vi "Compressor Rig PC Main.vi"() -> ()   [LabVIEW 2018]
uses:
  type defs/rigStatusCluster.ctl
  type defs/UI loop data.ctl
  type defs/event data.ctl
  supporting VIs/polymorphic VIs/enqueue for message handler.vi
  supporting VIs/polymorphic VIs/enqueue for comms.vi
  supporting VIs/polymorphic VIs/enqueue for file IO.vi
  supporting VIs/polymorphic VIs/de-queue for user interface.vi
  supporting VIs/polymorphic VIs/release user interface queue.vi
  RT/Message Handler loop/FPGA commands/RT - FPGA commands.lvlib
panel:
  in  "startPulsator":bool
  out "pulsatorHome":bool caption="Home"
  out "pulsatorSpeed":i32 caption="Actual:" min=0 max=65
  in  "pulsatorSetpoint":i32 caption="Target:" min=0 max=5000
  out "Interlocks":T1
  in  "openValves":bool
  in  "ballDemand":dbl caption="Ball Valve (%)" min=0.0 max=100.0 format="%_3g"
  in  "butterflyDemand":dbl=100.0 caption="Butterfly Valve (%)" min=0.0 max=100.0 format="%_3g"
  out "actualBall":dbl caption="Ball position" format="%_3f"
  out "actualButterfly":dbl caption="Butterfly position" format="%_3f"
  out "PR":dbl caption="Pressure Ratio" format="%_4f"
  out "massFlow":dbl caption="Mass Flow (kg/s)" format="%_4f"
  in  "logLimitEnabled":bool caption="limit logging"
  in  "pointLimit":u32 caption="datapoints"
  in  "timeLimit":dbl caption="log time (s)"
  in  "logData":bool
  out "speedGauge":dbl(knob) scale=0.0..75.0
  in  "targetSpeed":dbl caption="Target Speed (kRPM):" min=0.0 max=80.0 step=0.1 format="%_4g"
  in  "motorStart":bool
  out "statusCluster":T2 {"outletTemp" scale=0.0..100.0; "bearingTemp" scale=0.0..100.0; "gearboxTemp" scale=0.0..100.0}
  out "connected":bool caption="Compressor Rig Connected"
  in  "QUIT":bool
  # "Pulsator"
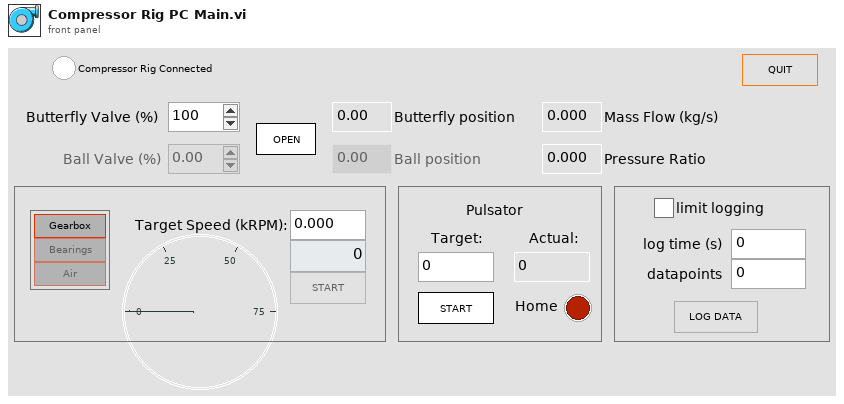
[diagram p1: front panel]
types:
  T1 = cluster{"gearboxOil":bool, "bearingOil":bool, "gearboxAir":bool}
  T2 = typedef "rigStatusCluster.ctl" = cluster{"water":bool, "airPressure":bool, "motorEnabled":bool, "oilPressure":bool, "outletTemp":dbl, "bearingTemp":dbl, "gearboxTemp":dbl}
  T3 = typedef "event data.ctl" = cluster{"menuRef":refnum<k9>, "channelConfigPath":path, "tempOffsets":dbl[]}
  T4 = typedef "UI loop data.ctl" = cluster{"params":cluster{"channelConfigPath":path, "version":string}, "vars":cluster{"tempOffsets":dbl[], "encoderFallingEdge":bool, "controlRefs":cluster{"mainVI":refnum<vi>, "menu":refnum<k9>, "motorStart":refnum<vi>, "butterfly":refnum<vi>, "ball":refnum<vi>, "speed":refnum<vi>, "logLimit":refnum<vi>, "pointLimit":refnum<vi>, "logData":refnum<vi>}}}
  T5 = typedef "message handler data.ctl" = cluster{"params":cluster{"configFileID":u32, "configFilePath":path, "channelConfigFilePath":path, "incidentLogfile":path, "controlChannels":cluster{"ballControl":u16, "butterflyControl":u16, "speedControl":u16}, "pulsatorVIPath":path, "customVIPath":path, "HowdenAir":cluster{"vent Howden":bool, "Howden%":dbl}}, "vars":cluster{"commsStatus":bool[], "controlIndex":cluster{"ballControl":u16, "butterflyControl":u16, "speedControl":u16}, "customVIRef":refnum<vi>, "Interlocks":cluster{"gearboxOil":bool, "bearingOil":bool, "gearboxAir":bool}, "motorRunning":bool, "liveDataQ":refnum<queue>[]}}
  T6 = typedef "comms loop data.ctl" = cluster{"params":cluster{"commandStream":cluster{"reader name":string, "writer name":string, "stream buffer size":i32}, "errorStream":cluster{"reader name":string, "writer name":string, "stream buffer size":i32}, "RT IP address":string, "pulserControllerIP":string}, "vars":cluster{"commandStream":refnum<k21>, "Incident logger":refnum<class "Incident logger.lvclass">, "check error scheduled message":u32, "errorStream":refnum<k21>, "watchdogScheduleID":u32, "pulsator":cluster{"pulser connection":refnum<class "Modbus Master.lvclass">, "pulserConnected":bool, "pulsatorScheduleID":u32, "pulserRunning":bool}}}
  T7 = typedef "data stream data.ctl" = cluster{"params":cluster{"Stream":cluster{"reader name":string, "RT IP address":string, "writer name":string, "stream buffer size":i32}}, "vars":cluster{"data stream":refnum<k21>}}
  T8 = typedef "data processor data.ctl" = cluster{"params":cluster{"controlFeedback":cluster{"butterflyValue":u16, "ballValue":u16, "massflow":u16, "pressureRatio":u16, "compSpeed":u16}, "DAQrate":enum16{"50 kHz", "25 kHz", "16.6 kHz", "12.5 kHz", "10 kHz", "8.33 kHz", "7.14 kHz", "6.25 kHz", "5.55 kHz", "5 kHz"}, "safetyChannels":cluster{"oilP":u16, "airP":u16, "water":u16, "channelLimit":T9[]}, "channelConfigPath":path}, "vars":cluster{"controlFeedback":cluster{"butterflyValue":u16, "ballValue":u16, "massflow":u16, "pressureRatio":u16, "compSpeed":u16}, "activeChannelNames":string[], "activeChannelUnits":string[], "offset trigger":bool, "offsets":dbl[], "activeChannelLimitIndex":u16[], "liveData":bool}}
  T9 = typedef "channelLimitControl.ctl" = cluster{"channelID":u16, "Enabled":bool, "warnValue":dbl, "limitValue":dbl, "Invert":bool, "limitAction":T10}
  T10 = typedef "limitActions.ctl" = enum16{"stop", "shutdown", "ignore"}
  T11 = typedef "file IO data.ctl" = cluster{"params":cluster{"startFolder":path, "channelConfigPath":path}, "vars":cluster{"channelConfig ":T12[], "writing":cluster{"streaming":bool, "fixedLength":bool, "pointCount":u32, "timeZero":dbl, "pointsWritten":u32, "dataRate":u16}, "channelCount":u16, "fileTarget":cluster{"Save folder":path, "Target filename":string, "file ref":refnum<file>, "pulsatorSpeed":string, "motorSpeed":string, "valvePosition":string, "torqueFilter":bool, "pulsatorRunning":bool, "motorRunning":bool}, "channels":refnum<class "Data Channel.lvclass">[]}}
  T12 = typedef "channelControl.ctl" = cluster{"index":u16, "active":bool, "channelType":T13, "module":u16, "terminal":u16, "channelName":string, "scalingMethod":T14, "scalingParameters":dbl[], "scaledUnits":string, "tempOffset":dbl}
  T13 = typedef "channelScalingTypes.ctl" = enum16{"calculation", "measurement", "scanivalve", "output", "digital"}
  T14 = typedef "scalingMethods.ctl" = enum16{"none", "linear", "thermocouple", "polynomial", "encoder", "RTD"}
  T15 = typedef "error messages data.ctl" = cluster{"params":cluster{"eg":bool}, "vars":cluster{"eg":bool}}
  T16 = cluster{"messageHandler":T5, "comms":T6, "dataStream":T7, "dataProcessor":T8, "fileIO":T11, "userInterface":T4, "errors":T15}
  T17 = typedef "Queues.ctl" = cluster{"messageHandler":refnum<queue>, "comms":refnum<queue>, "dataStream":refnum<queue>, "dataProcessor":refnum<queue>, "fileIO":refnum<queue>, "userInterface":refnum<queue>, "errors":refnum<queue>, "customCompressor":refnum<queue>}
  T18 = enum8{"Enabled", "Disabled", "Disabled and Grayed Out"}
  T19 = cluster{"actualSpeed":dbl, "butterfly":dbl, "ball":dbl, "massflow":dbl, "PR":dbl}
  T20 = typedef "eventvkey.ctl" = enum16{"ASCII", "Enter", "Return", "Shift", "Ctrl", "Alt", "Cmd", "Opt", "Caps", "NumLock", "Clear", "Break", "Up", "Down", "Left", "Right", "Insert", "Delete", "Home", "End", "PageUp", "PageDown", "Escape", "Help", "Pause", "ScrollLock", "F1", "F2", "F3", "F4", "F5", "F6", "F7", "F8", "F9", "F10", "F11", "F12", "F13", "F14", "F15", "F16", "F17", "F18", "F19", "F20", "F21", "F22", "F23", "F24", "Play", "VolumeUp", "VolumeDown", "Mute", "Two Byte Char"}
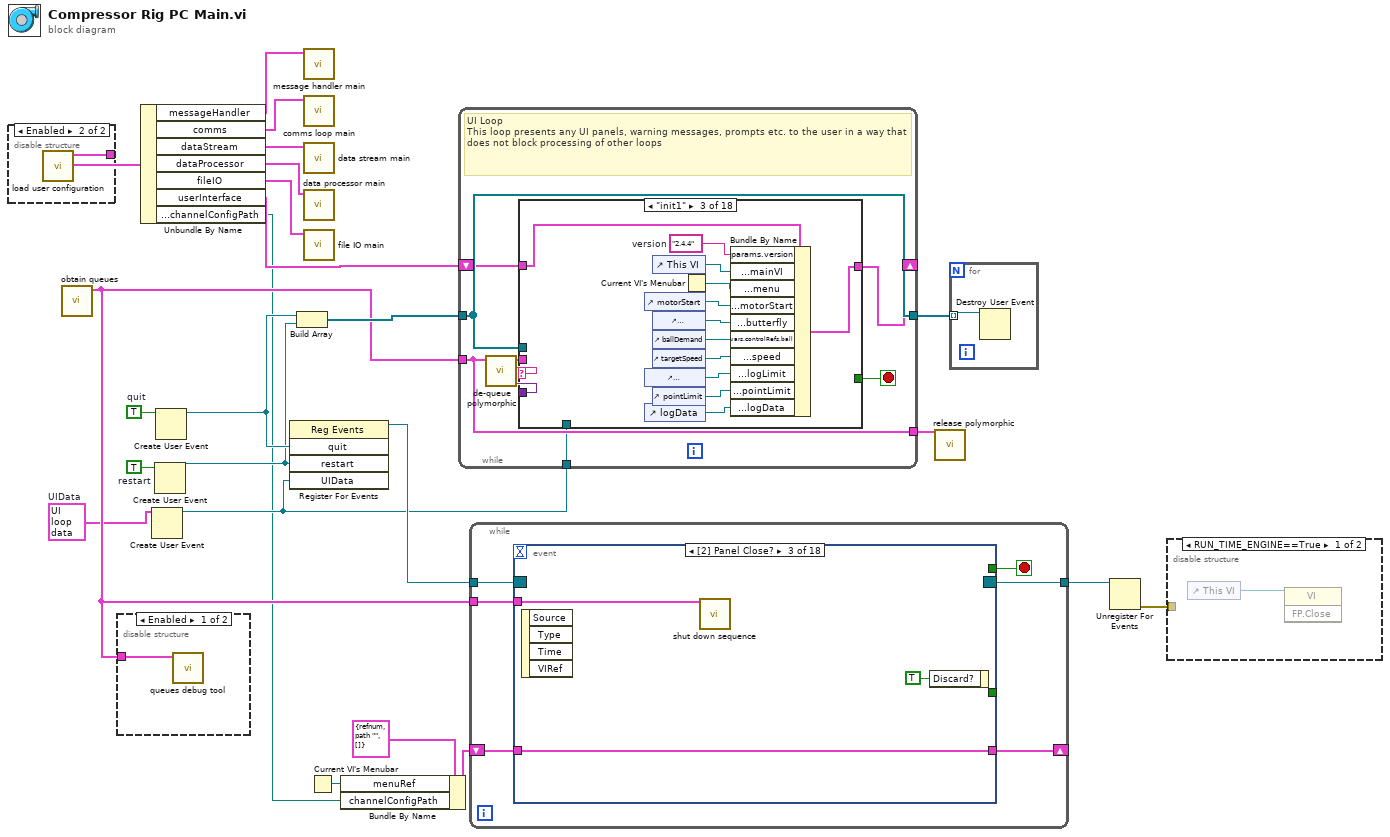
[diagram p0: block diagram]
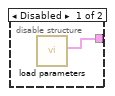
[diagram p4: hidden frame]
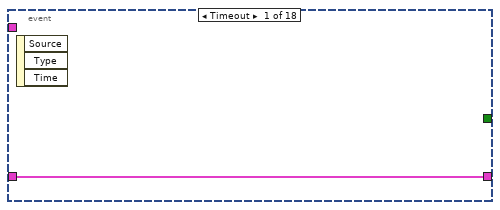
[diagram p5: hidden frame]
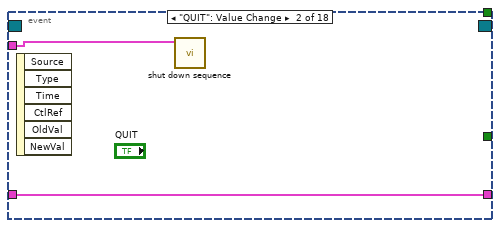
[diagram p6: hidden frame]
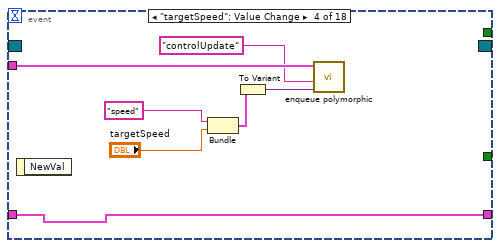
[diagram p7: hidden frame]
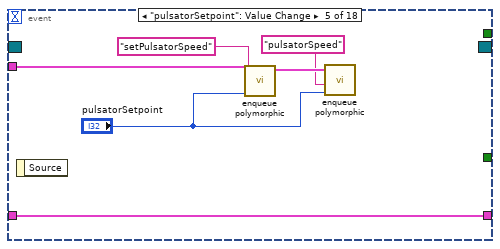
[diagram p8: hidden frame]
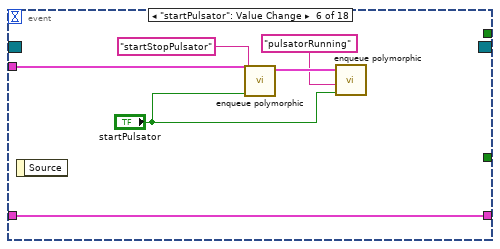
[diagram p9: hidden frame]
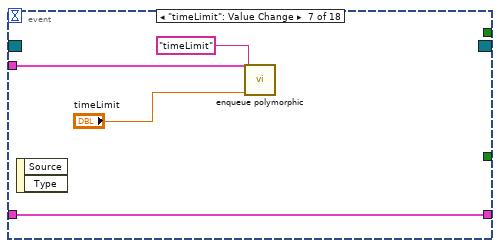
[diagram p10: hidden frame]
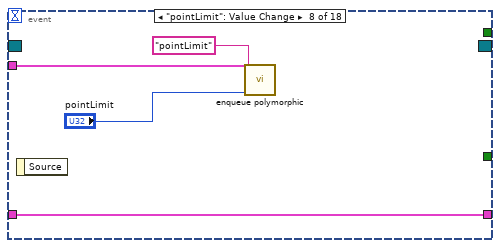
[diagram p11: hidden frame]
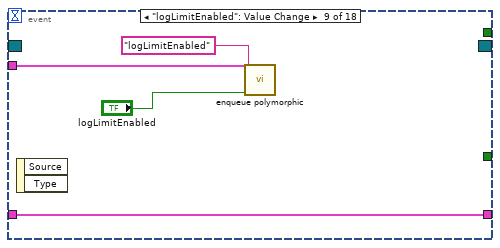
[diagram p12: hidden frame]
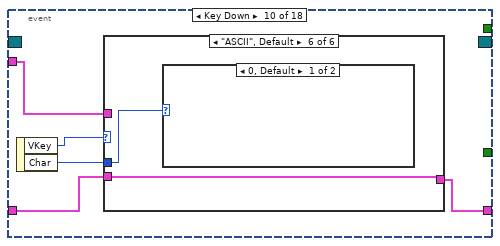
[diagram p13: hidden frame]
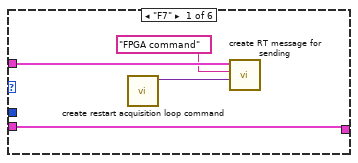
[diagram p14: hidden frame]
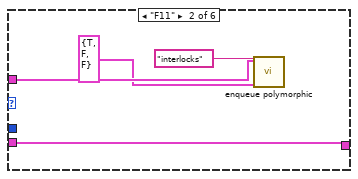
[diagram p15: hidden frame]
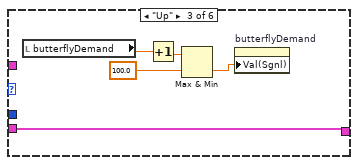
[diagram p16: hidden frame]
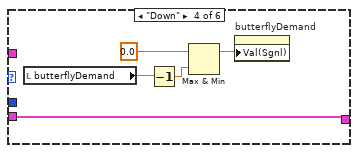
[diagram p17: hidden frame]
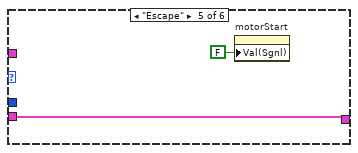
[diagram p18: hidden frame]
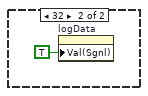
[diagram p19: hidden frame]
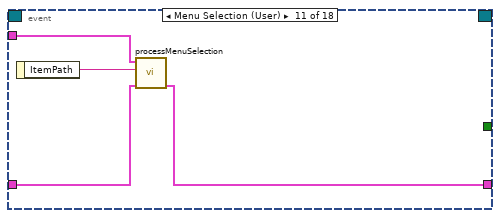
[diagram p20: hidden frame]
diagram:
  w7 = T4 {"params"={"channelConfigPath"=path "", "version"=""}, "vars"={"tempOffsets"=[], "encoderFallingEdge"=FALSE, "controlRefs"={"mainVI"=refnum, "menu"=refnum, "motorStart"=refnum, "butterfly"=refnum, "ball"=refnum, "speed"=refnum, "logLimit"=refnum, "pointLimit"=refnum, "logData"=refnum}}}  # UIData
  w12 = TRUE  # restart
  w20 = TRUE  # quit
  n1 = disable-structure shown="Enabled" {
    disable-tunnel: [w25 w26] -> w15
    frame Disabled {
      n2 = call "load parameters.vi"() -> ("parameters"=w25:T16)  [unwired: 11 in]
    }
    frame Enabled {
      n3 = call "load user configuration.vi"() -> ("config parameters"=w26:T16)  [unwired: 10 in, 1 out]
    }
  }
  n4 = call "obtain queues.vi"() -> ("queues"=w8:T17)  [unwired: 11 in]
  n5 = disable-structure shown="Enabled" {
    disable-tunnel: w8 -> [w27 _]
    frame Enabled {
      n6 = call "queues debug tool.vi"("queues"=w27) -> ()  [unwired: 11 in]
    }
    frame Disabled {
    }
  }
  n7 = Unbundle By Name(w15) -> ("messageHandler"=w14:T5, "comms"=w23:T6, "dataStream"=w24:T7, "dataProcessor"=w22:T8, "fileIO"=w21:T11, "userInterface"=w2:T4, "userInterface.params.channelConfigPath"=w1:path)
  n8 = Create User Event(user event datatype=w7) -> (user event=w6:refnum<user-event>)  [unwired: 1 in, 1 out]
  n9 = Create User Event(user event datatype=w12) -> (user event=w10:refnum<user-event>)  [unwired: 1 in, 1 out]
  n10 = Create User Event(user event datatype=w20) -> (user event=w17:refnum<user-event>)  [unwired: 1 in, 1 out]
  n11 = register-events(w17, w10, w6) -> (reference out=w19:refnum<event-registration>)  [unwired: 2 in, 1 out]
  n12 = Build Array(w17, w10) -> (w11:refnum<user-event>[])
  n13 = call "message handler main.vi"("messageHandler"=w14) -> ()  [unwired: 11 in]
  n14 = call "comms loop main.vi"("comms"=w23) -> ()  [unwired: 11 in]
  n15 = call "data stream main.vi"("dataStream"=w24) -> ()  [unwired: 11 in]
  n16 = call "data processor main.vi"("dataProcessor"=w22) -> ()  [unwired: 11 in]
  n17 = call "file IO main.vi"("fileIO"=w21) -> ()  [unwired: 11 in]
  n18 = Current VI's Menubar() -> (w3:refnum<k9>)
  n19 = Bundle By Name(cluster=T3 {"menuRef"=refnum, "channelConfigPath"=path "", "tempOffsets"=[]}, "menuRef"=w3, "channelConfigPath"=w1) -> (w4:T3)
  n20 = while {
    tunnel: w8 -> [w29]
    tunnel: w11 -> [w32]
    tunnel: [w32] -> w16
    shift-right: [w30] -> _
    shift-left: w2 -> [w31]
    tunnel: [w29] -> w9
    tunnel: w6 -> [w28]
    stop <- w33 stop-if-true
    # "UI Loop\nThis loop presents any UI panels, warning messages, prompts etc. to the user in a way that does not block processing of other loops"
    n21 = call-poly "de-queue polymorphic.vi"("Queues"=w29) -> ("data"=w34:variant, "message"=w35:string, "Queues out"=w36:T17)  [unwired: 8 in]
    n22 = case shown="\"init1\"" w35 {
      selector: w35 -> [w37 _ _ _ _ _ _ _ _ _ _ _ _ _ _ _ _ _]
      tunnel: w36 -> [w38 _ _ _ _ _ _ _ _ _ _ _ _ _ _ _ _ _]
      tunnel: w34 -> [_ _ _ w63 w66 w70 _ w79 w81 w88 w96 w101 _ w106 w117 w127 _ _]
      tunnel: [FALSE _ _ _ _ _ w74 _ _ _ _ _ _ _ _ _ _ _] -> w33
      tunnel: w32 -> [_ _ _ _ _ _ w75 _ _ _ _ _ _ _ _ _ _ w137]
      tunnel: w31 -> [w39 w42 w48 w61 w64 w67 w71 w76 w80 w85 w90 w98 w102 w108 w109 w118 w132 w133]
      tunnel: [w39 w42 w47 w61 w64 w67 w71 w76 w80 w85 w90 w98 w102 w108 w109 w118 w132 w133] -> w30
      tunnel: w28 -> [_ _ _ _ _ _ _ _ _ _ _ _ _ _ _ _ _ _]
      frame "", Default {
        n23 = call "unhandled message received.vi"("unhandledMessage"=w37, "queues"=w38) -> ()  [unwired: 10 in]
      }
      frame "init2" {
        n24 = flat-sequence {
          tunnel: w42 -> [w44]
          tunnel: [w44] -> w41
          tunnel: w41 -> [w45]
          frame #0 {
            n25 = Wait (ms)(milliseconds to wait=u32 250) -> ()  [unwired: 1 out]
          }
          frame #1 {
            n26 = call "set window title version.vi"("userInterface"=w45) -> ()  [unwired: 11 in]
          }
        }
      }
      frame "init1" {
        w49 = "2.4.4"  # version
        n27 = control-ref of="motorStart"() -> (w57:refnum<vi>)
        n28 = control-ref of="logLimitEnabled"() -> (w53:refnum<vi>)
        n29 = control-ref of="logData"() -> (w46:refnum<vi>)
        n30 = control-ref of="This VI"() -> (w51:refnum<vi>)
        n31 = control-ref of="butterflyDemand"() -> (w56:refnum<vi>)
        n32 = control-ref of="ballDemand"() -> (w55:refnum<vi>)
        n33 = control-ref of="targetSpeed"() -> (w54:refnum<vi>)
        n34 = control-ref of="pointLimit"() -> (w52:refnum<vi>)
        n35 = Current VI's Menubar() -> (w50:refnum<k9>)
        n36 = Bundle By Name(cluster=w48, "params.version"=w49, "vars.controlRefs.mainVI"=w51, "vars.controlRefs.menu"=w50, "vars.controlRefs.motorStart"=w57, "vars.controlRefs.butterfly"=w56, "vars.controlRefs.ball"=w55, "vars.controlRefs.speed"=w54, "vars.controlRefs.logLimit"=w53, "vars.controlRefs.pointLimit"=w52, "vars.controlRefs.logData"=w46) -> (w47:T4)
      }
      frame "howdenSettings" {
        n37 = Variant To Data(type=TRUE, Variant=w63) -> (data=w59:bool)  [unwired: 1 in, 1 out]
        n38 = Unbundle By Name(w61) -> ("vars.controlRefs.menu"=w62:refnum<k9>)
        n39 = Set Menu Item Info(6:w59, 7:"vent" ("item tag"), 11:w62) -> ()  [unwired: 4 in, 2 out]
      }
      frame "timeLimit" {
        n40 = Variant To Data(Variant=w66) -> (data=w65:dbl)  [unwired: 2 in, 1 out]
        n41 = local write "timeLimit"(w65) -> ()
      }
      frame "pointLimit" {
        n42 = Variant To Data(type=u32 0, Variant=w70) -> (data=w68:u32)  [unwired: 1 in, 1 out]
        n43 = local write "pointLimit"(w68) -> ()
      }
      frame "quit" {
        w74 = TRUE
        n44 = Index Array(array=w75) -> (element=w72:refnum<user-event>)  [unwired: 1 in]
        n45 = Generate User Event(user event=w72, event data cluster=w74) -> ()  [unwired: 2 in, 2 out]
        n46 = local write "connected"(FALSE ("connected")) -> ()
      }
      frame "connection status" {
        n47 = Variant To Data(type=TRUE ("connected"), Variant=w79) -> (data=→"connected":bool)  [unwired: 1 in, 1 out]
      }
      frame "rigStatus update" {
        n48 = disable-structure shown="Disabled" {
          disable-tunnel: w81 -> [w84 _]
          frame Disabled {
            n49 = Variant To Data(type=T2 {"water"=FALSE, "airPressure"=FALSE, "motorEnabled"=FALSE, "oilPressure"=FALSE, "outletTemp"=0.0, "bearingTemp"=0.0, "gearboxTemp"=0.0} ("statusCluster"), Variant=w84) -> (data=→"statusCluster":T2)  [unwired: 1 in, 1 out]
          }
          frame Enabled {
          }
        }
      }
      frame "userMessage" {
        n50 = Variant To Data(type="", Variant=w88) -> (data=w87:string)  [unwired: 1 in, 1 out]
        n51 = One Button Dialog(message=w87) -> ()  [unwired: 1 in, 1 out]
      }
      frame "interlocks" {
        n52 = Variant To Data(Variant=w96) -> (data=w95:T1)  [unwired: 2 in, 1 out]
        "Interlocks" <- w95
        n53 = Unbundle By Name(w90) -> ("vars.controlRefs.motorStart"=w89:refnum<vi>)
        n54 = call "check interlock status.vi"("Interlocks"=w95) -> ("interlocksOK"=w94:bool)  [unwired: 10 in]
        n55 = Select(t=T18."Enabled" ("Disabled"), s=w94, f=T18."Disabled and Grayed Out" ("Disabled")) -> (s? t:f=w91:T18)
        n56 = property class="Bool (strict)"(reference=w89, "DisabledEnum"=w91) -> ()  [unwired: 1 in, 2 out]
      }
      frame "motorStart" {
        n57 = Variant To Data(type=TRUE ("quit"), Variant=w101) -> (data=w100:bool)  [unwired: 1 in, 1 out]
        n58 = Unbundle By Name(w98) -> ("vars.controlRefs.motorStart"=w97:refnum<vi>)
        n59 = property class="Bool (strict)"(reference=w97, "Value"=w100) -> ()  [unwired: 1 in, 2 out]
      }
      frame "writeComplete" {
        n60 = local write "logData"(FALSE ("logData")) -> ()
      }
      frame "lastFile" {
        n61 = Unbundle By Name(w108) -> ("vars.controlRefs.logData"=w107:refnum<vi>)
        n62 = Variant To Data(type="", Variant=w106) -> (data=w104:string)  [unwired: 1 in, 1 out]
        n63 = property class="Bool (strict)"(reference=w107, "TipStrip"=w104) -> ()  [unwired: 1 in, 2 out]
      }
      frame "indicatorsUpdate" {
        n64 = Variant To Data(type=T19 {"actualSpeed"=0.0, "butterfly"=0.0, "ball"=0.0, "massflow"=0.0, "PR"=0.0} ("indicators"), Variant=w117) -> (data=w116:T19)  [unwired: 1 in, 1 out]
        n65 = Unbundle By Name(w116) -> ("actualSpeed"=→"speedGauge":dbl, "butterfly"=→"actualButterfly":dbl, "ball"=→"actualBall":dbl, "massflow"=→"massFlow":dbl, "PR"=→"PR":dbl)
      }
      frame "pulsatorUpdate" {
        n66 = Variant To Data(type=cluster{"poition":i32, "velocity":i32} {"poition"=0, "velocity"=0} ("pulsator state"), Variant=w127) -> (data=w125:cluster{"poition":i32, "velocity":i32})  [unwired: 1 in, 1 out]
        n67 = Unbundle By Name(w125) -> ("poition"=w121:i32, "velocity"=→"pulsatorSpeed":i32)
        n68 = In Range and Coerce(upper limit=355, x=w121, lower limit=5) -> (In Range?=w120:bool)  [unwired: 1 out]
        n69 = Not(x=w120) -> (.not. x?=→"pulsatorHome":bool)
      }
      frame "motor stop" {
        n70 = Unbundle By Name(w132) -> ("vars.controlRefs.motorStart"=w131:refnum<vi>, "vars.controlRefs.butterfly"=w129:refnum<vi>)
        n71 = property class="DigNum (strict)"(reference=w129, "Val(Sgnl)"=100.0 ("Value")) -> ()  [unwired: 1 in, 2 out]
        n72 = property class="Bool (strict)"(reference=w131, "Value"=FALSE) -> ()  [unwired: 1 in, 2 out]
      }
      frame "restart" {
        w136 = TRUE  # event data
        n73 = Index Array(array=w137, index=1) -> (element=w135:refnum<user-event>)
        n74 = Generate User Event(user event=w135, event data cluster=w136) -> ()  [unwired: 2 in, 2 out]
      }
    }
  }
  n75 = while {
    tunnel: w8 -> [w143]
    tunnel: w19 -> [w142]
    tunnel: [w140] -> w18
    shift-right: [w138] -> _
    shift-left: w4 -> [w139]
    stop <- w141 stop-if-true
    n76 = event shown="[2] Panel Close?" {
      selector: w142 -> [_ _ _ _ _ _ _ _ _ _ _ _ _ _ _ _ _ _]
      dyn-events: [_ _ _ _ _ _ _ _ _ _ _ _ _ _ _ _ _ _] -> w140
      timeout: _ -> [_ _ _ _ _ _ _ _ _ _ _ _ _ _ _ _ _ _]
      tunnel: w143 -> [_ w145 w148 w156 w162 w168 w172 w176 w180 w184 w211 w219 w226 w238 w244 w250 w252 _]
      tunnel: [_ _ _ _ _ _ _ _ _ _ _ _ _ _ _ _ _ TRUE] -> w141
      tunnel: w139 -> [w144 w146 w147 w150 w157 w166 w169 w173 w177 w183 w210 w213 w220 w234 w243 w245 w256 w258]
      tunnel: [w144 w146 w147 w150 w157 w166 w169 w173 w177 w182 w209 w213 w220 w234 w243 w245 w256 w258] -> w138
      tunnel: [_ _ _ _ _ _ _ _ _ _ _ _ _ "openValves" _ _ _ _] -> _
      event Timeout {
        n77 = event-data() -> ()  [unwired: 1 in, 3 out]
      }
      event "QUIT": Value Change {
        n78 = event-data() -> ()  [unwired: 1 in, 6 out]
        n79 = call "shut down sequence.vi"("queues"=w145) -> ()  [unwired: 11 in]
      }
      event Panel Close? {
        n80 = event-data() -> ()  [unwired: 1 in, 4 out]
        n81 = call "shut down sequence.vi"("queues"=w148) -> ()  [unwired: 11 in]
        n82 = event-data("Discard?"=TRUE) -> ()  [unwired: 1 in, 1 out]
      }
      event "targetSpeed": Value Change {
        n83 = event-data() -> ()  [unwired: 1 in, 1 out]
        n84 = Bundle("speed", "targetSpeed"="targetSpeed") -> (w153:cluster{string, "targetSpeed":dbl})  [unwired: 1 in]
        n85 = To Variant(anything=w153) -> (Variant=w152:variant)
        n86 = call-poly "enqueue polymorphic.vi"("data"=w152, "message"="controlUpdate", "Queues"=w156) -> ()  [unwired: 8 in, 1 out]
      }
      event "pulsatorSetpoint": Value Change {
        n87 = event-data() -> ()  [unwired: 1 in, 1 out]
        n88 = call-poly "enqueue polymorphic.vi"("data"="pulsatorSetpoint", "message"="setPulsatorSpeed", "Queues"=w162) -> ("Queues out"=w160:T17)  [unwired: 8 in]
        n89 = call-poly "enqueue polymorphic.vi"("data"="pulsatorSetpoint", "message"="pulsatorSpeed", "Queues"=w160) -> ()  [unwired: 8 in, 1 out]
      }
      event "startPulsator": Value Change {
        n90 = event-data() -> ()  [unwired: 1 in, 1 out]
        n91 = call-poly "enqueue polymorphic.vi"("data"="startPulsator", "message"="startStopPulsator", "Queues"=w168) -> ("Queues out"=w165:T17)  [unwired: 8 in]
        n92 = call-poly "enqueue polymorphic.vi"("data"="startPulsator", "message"="pulsatorRunning", "Queues"=w165) -> ()  [unwired: 8 in, 1 out]
      }
      event "timeLimit": Value Change {
        n93 = event-data() -> ()  [unwired: 1 in, 2 out]
        n94 = call-poly "enqueue polymorphic.vi"("data"="timeLimit", "message"="timeLimit", "Queues"=w172) -> ()  [unwired: 8 in, 1 out]
      }
      event "pointLimit": Value Change {
        n95 = event-data() -> ()  [unwired: 1 in, 1 out]
        n96 = call-poly "enqueue polymorphic.vi"("data"="pointLimit", "message"="pointLimit", "Queues"=w176) -> ()  [unwired: 8 in, 1 out]
      }
      event "logLimitEnabled": Value Change {
        n97 = event-data() -> ()  [unwired: 1 in, 2 out]
        n98 = call-poly "enqueue polymorphic.vi"("data"="logLimitEnabled", "message"="logLimitEnabled", "Queues"=w180) -> ()  [unwired: 8 in, 1 out]
      }
      event Key Down {
        n99 = event-data() -> ("VKey"=w185:T20, "Char"=w181:i16)  [unwired: 1 in]
        n100 = case shown="\"ASCII\", Default" w185 {
          tunnel: w184 -> [w189 w192 _ _ _ _]
          tunnel: [w186 w193 w198 w203 w205 w207] -> w182
          tunnel: w183 -> [w186 w193 w198 w203 w205 w207]
          tunnel: w181 -> [_ _ _ _ _ w206]
          frame "F7" {
            n101 = call "create restart acquisition loop command.vi"() -> ("command message"=w188:variant)  [unwired: 11 in]
            n102 = call "create RT message for sending.vi"("RT data"=w188, "RT message"="FPGA command", "Queues in"=w189) -> ()  [unwired: 8 in, 1 out]
          }
          frame "F11" {
            n103 = call-poly "enqueue polymorphic.vi"("data"=T1 {"gearboxOil"=TRUE, "bearingOil"=FALSE, "gearboxAir"=FALSE} ("vars.Interlocks"), "message"="interlocks", "Queues"=w192) -> ()  [unwired: 8 in, 1 out]
          }
          frame "Up" {
            n104 = local read "butterflyDemand"() -> (w194:dbl)
            n105 = Increment(x=w194) -> (x+1=w195:dbl)
            n106 = Max & Min(x=w195, y=100.0) -> (min(x,y)=w196:dbl)  [unwired: 1 out]
            n107 = property on="butterflyDemand" class="DigNum (strict)"("Val(Sgnl)"=w196) -> ()  [unwired: 2 in, 2 out]
          }
          frame "Down" {
            n108 = local read "butterflyDemand"() -> (w200:dbl)
            n109 = Decrement(x=w200) -> (x-1=w199:dbl)
            n110 = Max & Min(x=0.0, y=w199) -> (max(x,y)=w201:dbl)  [unwired: 1 out]
            n111 = property on="butterflyDemand" class="DigNum (strict)"("Val(Sgnl)"=w201) -> ()  [unwired: 2 in, 2 out]
          }
          frame "Escape" {
            n112 = property on="motorStart" class="Bool (strict)"("Val(Sgnl)"=FALSE ("Value (Signaling)")) -> ()  [unwired: 2 in, 2 out]
          }
          frame "ASCII", Default {
            n113 = case shown="0, Default" w206 {
              frame 0, Default {
              }
              frame 32 {
                n114 = property on="logData" class="Bool (strict)"("Val(Sgnl)"=TRUE ("Value (Signaling)")) -> ()  [unwired: 2 in, 2 out]
              }
            }
          }
        }
      }
      event Menu Selection (User) {
        n115 = event-data() -> ("ItemPath"=w212:string)  [unwired: 1 in]
        n116 = call "processMenuSelection.vi"("eventData"=w210, "ItemPath"=w212, "queues"=w211) -> ("eventData 2"=w209:T3)  [unwired: 8 in]
      }
      event "butterflyDemand": Value Change {
        n117 = event-data() -> ()  [unwired: 1 in, 1 out]
        n118 = Bundle("butterflyValve", "butterflyDemand"="butterflyDemand") -> (w216:cluster{string, "butterflyDemand":dbl})  [unwired: 1 in]
        n119 = To Variant(anything=w216) -> (Variant=w215:variant)
        n120 = call-poly "enqueue polymorphic.vi"("data"=w215, "message"="controlUpdate", "Queues"=w219) -> ()  [unwired: 8 in, 1 out]
      }
      event "ballDemand": Value Change {
        n121 = event-data() -> ()  [unwired: 1 in, 1 out]
        n122 = Bundle("ballValve", "ballDemand"="ballDemand") -> (w223:cluster{string, "ballDemand":dbl})  [unwired: 1 in]
        n123 = To Variant(anything=w223) -> (Variant=w222:variant)
        n124 = call-poly "enqueue polymorphic.vi"("data"=w222, "message"="controlUpdate", "Queues"=w226) -> ()  [unwired: 8 in, 1 out]
      }
      event "openValves": Value Change {
        w228 = 100.0
        w232 = "controlUpdate"
        n125 = event-data() -> ()  [unwired: 1 in, 1 out]
        n126 = Bundle("butterflyValve", w228) -> (w236:cluster{string, dbl})  [unwired: 1 in]
        n127 = To Variant(anything=w236) -> (Variant=w235:variant)
        n128 = call-poly "enqueue polymorphic.vi"("data"=w235, "message"=w232, "Queues"=w238) -> ("Queues out"=w233:T17)  [unwired: 8 in]
        n129 = Bundle("ballValve", w228) -> (w230:cluster{string, dbl})  [unwired: 1 in]
        n130 = local write "butterflyDemand"(w228) -> ()
        n131 = local write "ballDemand"(w228) -> ()
        n132 = To Variant(anything=w230) -> (Variant=w229:variant)
        n133 = call-poly "enqueue polymorphic.vi"("data"=w229, "message"=w232, "Queues"=w233) -> ()  [unwired: 8 in, 1 out]
      }
      event "motorStart": Value Change {
        w241 = "motorStart" ("message")
        n134 = event-data() -> ()  [unwired: 1 in, 1 out]
        n135 = To Variant(anything="motorStart") -> (Variant=w239:variant)
        n136 = call-poly "enqueue polymorphic.vi"("data"=w239, "message"=w241, "Queues"=w244) -> ("Queues out"=w242:T17)  [unwired: 8 in]
        n137 = call-poly "enqueue polymorphic.vi"("data"=w239, "message"=w241, "Queues"=w242) -> ()  [unwired: 8 in, 1 out]
      }
      event "logData": Value Change {
        n138 = event-data() -> ()  [unwired: 1 in, 1 out]
        n139 = Select(t="start" ("message"), s="logData", f="stop" ("message")) -> (s? t:f=w247:string)
        n140 = call-poly "enqueue polymorphic.vi"("message"=w247, "Queues"=w250) -> ()  [unwired: 9 in, 1 out]
      }
      event User Event {
        n141 = event-data() -> ()  [unwired: 1 in, 4 out]
        n142 = Two Button Dialog(message="You need to restart the controller to apply the changes.\nQuit Now?", 1:"Later" ("F button name (\"Cancel\")"), 2:"Quit Now" ("T button name (\"OK\")")) -> (T button?=w251:bool)
        n143 = case shown="True" w251 {
          tunnel: w252 -> [_ w257]
          frame False {
          }
          frame True {
            n144 = call "shut down sequence.vi"("queues"=w257) -> ()  [unwired: 11 in]
          }
        }
      }
      event User Event {
        n145 = event-data() -> ()  [unwired: 1 in, 5 out]
      }
    }
  }
  n146 = call-poly "release polymorphic.vi"("Queues"=w9) -> ()  [unwired: 11 in]
  n147 = for {
    tunnel: w16 -> [w260] mode=indexing
    n148 = Destroy User Event(user event=w260) -> ()  [unwired: 1 in, 1 out]
  }
  n149 = Unregister For Events(event registration refnum=w18) -> (error out=w13:errorcluster)  [unwired: 1 in]
  n150 = disable-structure shown="RUN_TIME_ENGINE==True" {
    disable-tunnel: w13 -> [_ _]
    frame condition #0 {
      n151 = control-ref of="This VI"() -> (w261:refnum<vi>)
      n152 = invoke class="VI" method="FP.Close"(reference=w261) -> ()  [unwired: 2 in, 3 out]
    }
    frame condition #1 (active) {
    }
  }
